vi "set_ref_clus_TPG361.vi"(6 "cluster_ref_TPG361":T1, 10 "PR1":dbl, 11 "status":bool) -> ()   [LabVIEW 2019]
uses:
  cluster_ref_TPG361.ctl
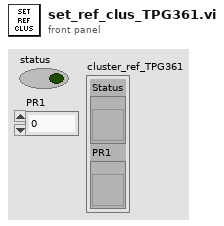
[diagram p1: front panel]
types:
  T1 = typedef "cluster_ref_TPG361.ctl" = cluster{"Status":refnum<vi>, "PR1":refnum<vi>}
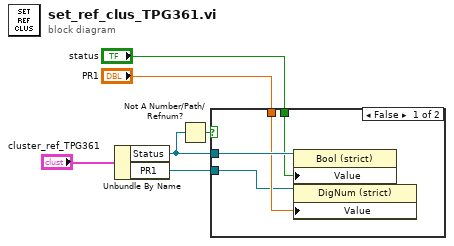
[diagram p0: block diagram]
diagram:
  n1 = Unbundle By Name("cluster_ref_TPG361") -> ("Status"=w5:refnum<vi>, "PR1"=w4:refnum<vi>)
  n2 = Not A Number/Path/Refnum?(number/path/refnum=w5) -> (NaN/Path/Refnum?=w6:bool)
  n3 = case shown="False" w6 {
    tunnel: w5 -> [w10 _]
    tunnel: w4 -> [w7 _]
    tunnel: "status" -> [w9 _]
    tunnel: "PR1" -> [w8 _]
    frame False {
      n4 = property class="Bool (strict)"(reference=w10, "Value"=w9) -> ()  [unwired: 1 in, 2 out]
      n5 = property class="DigNum (strict)"(reference=w7, "Value"=w8) -> ()  [unwired: 1 in, 2 out]
    }
    frame True {
    }
  }
